vi "LVClasse_Intensity Resize Data.vi"(0 "Intensity in":refnum<class "Intensity.lvclass">, 5 "Factor":u8, 7 "Intensity in":refnum<class "Intensity.lvclass">, 9 "do_erode":bool, 11 "error in (no error)":errorcluster) -> (4 "Intensity out":refnum<class "Intensity.lvclass">, 8 "Intensity in 2":refnum<class "Intensity.lvclass">, 15 "error out":errorcluster)   [LabVIEW 2020, in "Intensity.lvclass"]
doc: "Phase values buffer and pupil setter.\n\n--------------------------------------------------------------------------------\n\n<B>PhaseIn </B> : Phase object.\n<B>PhaseOut </B> : Phase object.\n<B>buffer </B> : Phase values buffer.\n<B>Pupil </B> : pupil object.\n<B>ErrorIn </B> : Error\n<B>ErrorOut </B> : Error\n\n--------------------------------------------------------------------------------"
uses:
  Intensity.lvclass
  Intensity.lvclass/Intensity.ctl
  LVClasse_Phase Read Intensity.vi
panel:
  out "?":u8
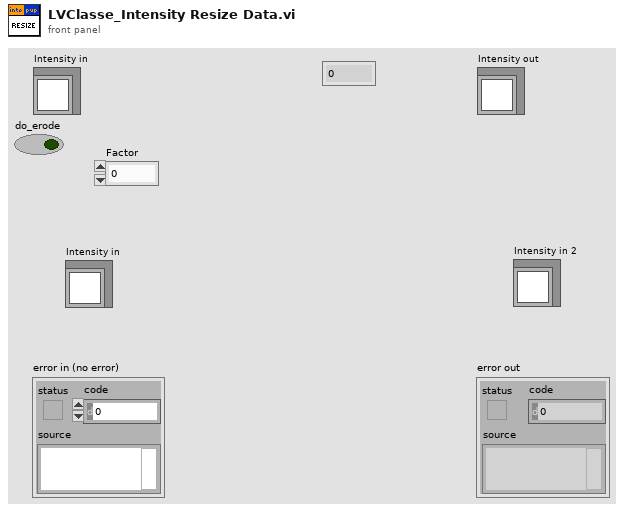
[diagram p1: front panel]
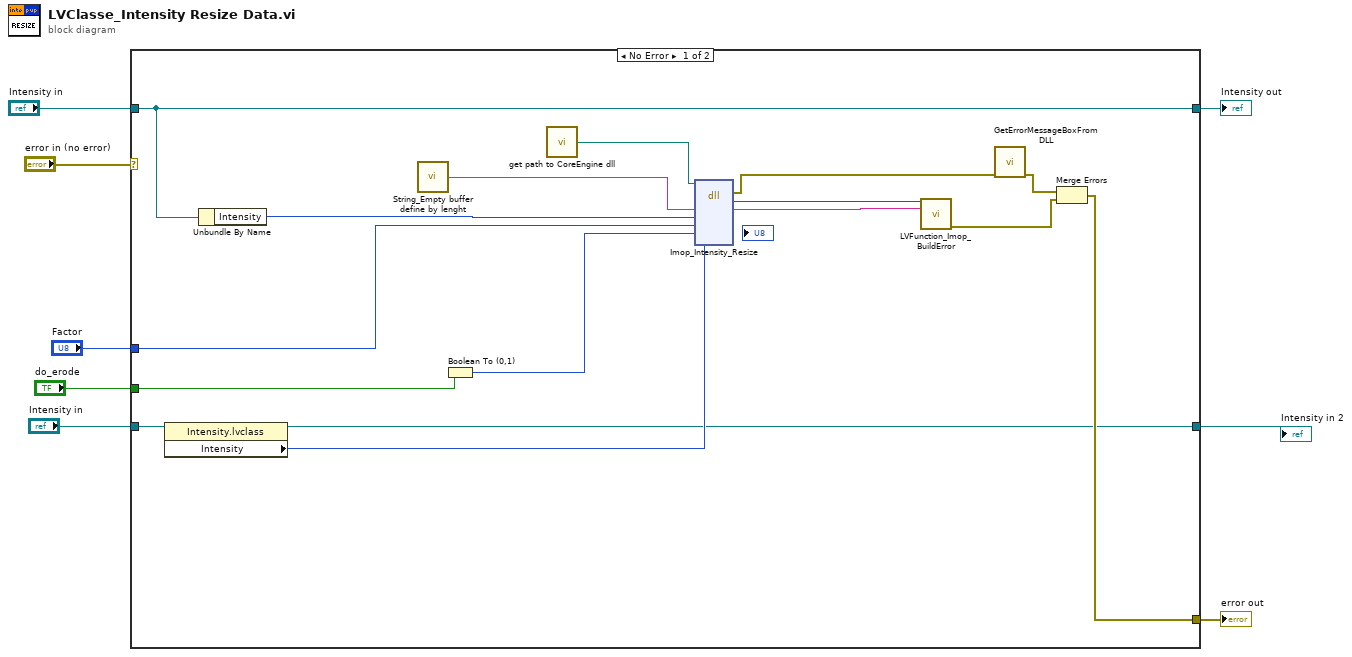
[diagram p0: block diagram]
diagram:
  n1 = case shown="No Error" "error in (no error)" {
    selector: "error in (no error)" -> [_ w27]
    tunnel: [w13 w27] -> w8
    tunnel: [w19 w26] -> w7
    tunnel: "Intensity in" -> [w19 w26]
    tunnel: "Intensity in" -> [w17 w25]
    tunnel: "Factor" -> [w12 _]
    tunnel: [w11 w25] -> w2
    tunnel: "do_erode" -> [w9 _]
    frame No Error {
      n2 = property class="Intensity.lvclass"(reference=w17) -> (reference out=w11:refnum<class "Intensity.lvclass">, "Intensity"=w16:i32)  [unwired: 1 in, 1 out]
      n3 = Unbundle By Name(w19) -> ("Intensity"=w18:i32)
      n4 = call "String_Empty buffer define by lenght.vi"() -> ("Empty buffer"=w22:string)  [unwired: 1 in]
      n5 = Boolean To (0,1)(Boolean=w9) -> (0, 1=w10:i16)
      n6 = call "get path to CoreEngine dll.vi"() -> ("path to c_interface_vc100.dll"=w21:path)  [unwired: 12 in, 3 out]
      n7 = dll-call lib="D:/2_trunk/Soft_haso/ImOpCoreEngine4_LV2011/DLLs/ImopEngine4_vc100.dll" fn="Imop_Intensity_Resize"(path in=w21, "message"=w22, "intensity"=w18, "factor"=w12, "do_erode"=w10, "resized pupil"=w16) -> (error out=w20:errorcluster, "return type"=w24:i32, "message"=w23:string)  [unwired: 6 in, 1 out]
      n8 = call "LVFunction_Imop_BuildError.vi"("code"=w24, "String to Prepend to source (\"\")"=w23) -> ("error out"=w14:errorcluster)  [unwired: 13 in]
      n9 = call "GetErrorMessageBoxFromDLL.vi"("error IN"=w20) -> ("error OUT"=w15:errorcluster)  [unwired: 10 in]
      n10 = Merge Errors(w15, w14) -> (w13:errorcluster)
    }
    frame Error {
    }
  }
  "error out" <- w8
  "Intensity out" <- w7
  "Intensity in 2" <- w2
